vi "FOCUS_V42_H37.vi"(9 "X-pixels":sgl=256.0, 11 "Run":bool) -> (0 "Retrace pixels":sgl, 10 "Pixel Clock (Hz)":sgl)   [LabVIEW 2010] (continued)
                frame 2 {
                  # "line scan FScope"
                  n3346 = local read "LS X/Y"() -> (w6475:bool)
                  n3347 = case shown="True" w6475 {
                    tunnel: [w6513 w6514] -> w6476
                    frame False {
                      n3348 = local read "Y dim"() -> (w6513:sgl)
                    }
                    frame True {
                      n3349 = local read "X dim"() -> (w6514:sgl)
                    }
                  }
                  n3350 = Initialize Array(u32 0 ("element"), w6476) -> (w6477:u32[])
                  n3351 = Unbundle By Name(w6497) -> ("status"=w6495:bool)
                  n3352 = Unbundle By Name(w6493) -> ("status"=w6492:bool)
                  n3353 = Unbundle By Name(w6496) -> ("status"=w6494:bool)
                  n3354 = while {
                    tunnel: w6506 -> [w6586]
                    tunnel: w6505 -> [w6585]
                    tunnel: [w6584] -> w6504
                    tunnel: [w6576] -> w6503
                    shift-right: [w6524] -> w6473
                    shift-left: w6498 -> [w6536]
                    shift-right: [w6526] -> w6472
                    shift-left: w6498 -> [w6535]
                    tunnel: [w6580] -> w6500
                    tunnel: w6502 -> [w6580]
                    tunnel: [w6577] -> w6499
                    tunnel: w6501 -> [w6577]
                    shift-right: [w6530] -> _
                    shift-left: w6477 -> [w6519]
                    tunnel: w6495 -> [w6573]
                    tunnel: w6494 -> [w6578]
                    tunnel: w6492 -> [w6561]
                    shift-right: [w6567] -> _
                    shift-left: sgl 0.0 ("millisecond timer value") -> [w6570]
                    tunnel: w6490 -> [w6566]
                    tunnel: w6487 -> [w6564]
                    tunnel: [w6564] -> w6485
                    tunnel: [w6563] -> w6484
                    tunnel: w6486 -> [w6563]
                    tunnel: w6483 -> [w6529]
                    shift-right: [w6551] -> _
                    shift-left: w6481 -> [w6553]
                    shift-right: [w6549] -> _
                    shift-left: w6482 -> [w6550]
                    tunnel: w6475 -> [w6533]
                    tunnel: [w6522] -> w6474
                    i -> [w6528]
                    stop <- w6572 stop-if-true
                    n3355 = local read "ScaleCluster"() -> (w6559:T3)
                    n3356 = local read "Overlay Images"() -> (w6581:bool)
                    n3357 = Bundle("ScaleCluster"=w6559, "scans to read"=w6529) -> (w6551:T20)  [unwired: 1 in]
                    n3358 = call-poly <vilib>:"DAQmx Read (Digital 1D U32 1Chan NSamp).vi"("task/channels in"=w6586, "number of samples per channel"=w6529, "error in"=w6585) -> ("task out"=w6584:refnum<k21>, "data"=w6517:u32[], "error out"=w6576:errorcluster)  [unwired: 10 in]
                    n3359 = Not Equal?(x=w6551, y=w6553) -> (x != y?=w6552:bool)
                    n3360 = Multiply(x=u32 0 ("millisecond timer value"), y=w6519) -> (x*y=w6518:u32[])
                    n3361 = call-poly <vilib>:"Ramp Pattern.vi"("start"=0.0, "end"=6.283185307179586, "samples"=w6529) -> ("Ramp Pattern"=w6548:dbl[])  [unwired: 7 in, 1 out]
                    n3362 = case shown="False" w6552 {
                      tunnel: w6566 -> [_ w6592]
                      tunnel: [w6589 w6591] -> w6549
                      tunnel: w6551 -> [_ w6590]
                      tunnel: w6550 -> [w6589 _]
                      frame False {
                      }
                      frame True {
                        n3363 = call "ScaleScanlineFScope.vi"("Parameters"=w6592, "ScaleCluster"=w6590) -> ("ScanlineScaled"=w6591:dbl[][])
                      }
                    }
                    n3364 = Split Number(x=w6517) -> (hi(x)=w6583:u16[])  [unwired: 1 out]
                    n3365 = Sine(x=w6548) -> (sin(x)=w6546:dbl[])
                    n3366 = Split Number(x=w6583) -> (hi(x)=w6521:u8[], lo(x)=w6582:u8[])
                    n3367 = case shown="True" w6581 {
                      tunnel: w6521 -> [w6598 w6617]
                      tunnel: [w6598 w6600] -> w6534
                      tunnel: w6582 -> [w6597 w6619]
                      tunnel: [w6597 _] -> w6531
                      frame False {
                      }
                      frame True {
                        n3368 = To Word Integer(number=w6617) -> (16bit integer=w6618:i16[])
                        n3369 = Subtract(x=w6618, y=w6619) -> (x-y=w6599:i16[])
                        n3370 = Add(x=w6618, y=w6619) -> (x+y=w6613:i16[])
                        n3371 = Increment(x=w6613) -> (x+1=w6623:i16[])
                        n3372 = Divide(x=w6599, y=w6623) -> (x/y=w6622:dbl[])
                        n3373 = Absolute Value(x=w6599) -> (abs(x)=w6615:i16[])
                        n3374 = Multiply(x=w6622, y=u8 2) -> (x*y=w6620:dbl[])
                        n3375 = Round To Nearest(number=w6620) -> (nearest integer value=w6606:dbl[])
                        n3376 = Divide(x=w6615, y=2.0) -> (x/y=w6612:dbl[])
                        n3377 = Divide(x=w6613, y=2.0) -> (x/y=w6611:dbl[])
                        n3378 = Add(x=w6612, y=w6611) -> (x+y=w6609:dbl[])
                        n3379 = Divide(x=w6609, y=5.0) -> (x/y=w6608:dbl[])
                        n3380 = Round To Nearest(number=w6608) -> (nearest integer value=w6607:dbl[])
                        n3381 = Multiply(x=5.0 ("y"), y=w6607) -> (x*y=w6605:dbl[])
                        n3382 = Add(x=w6606, y=w6605) -> (x+y=w6604:dbl[])
                        n3383 = Subtract(x=w6604, y=2.0) -> (x-y=w6601:dbl[])
                        n3384 = To Unsigned Byte Integer(number=w6601) -> (unsigned 8bit integer=w6600:u8[])
                      }
                    }
                    n3385 = Add(x=w6546, y=sgl 2.0 ("millisecond timer value")) -> (x+y=w6541:dbl[])
                    n3386 = Divide(x=u32 4294967295 ("millisecond timer value"), y=sgl 3.0) -> (x/y=w6542:sgl)
                    n3387 = Array Subset(array=w6549, index (col)=w6570, length (col)=w6529) -> (w6532:dbl[][])  [unwired: 2 in]
                    n3388 = Multiply(x=w6542, y=w6541) -> (x*y=w6540:dbl[])
                    n3389 = To Unsigned Long Integer(number=w6540) -> ()  [unwired: 1 out]
                    n3390 = Index Array(array=w6549, index (row)=0) -> (element=w6557:dbl[])  [unwired: 1 in]
                    n3391 = Array Size(array=w6557) -> (size(s)=w6555:i32)
                    n3392 = Divide(x=w6555, y=2) -> (x/y=w6554:dbl)
                    n3393 = Add(x=w6570, y=w6529) -> (x+y=w6568:dbl)
                    n3394 = local read "LS X/Y"() -> (w6538:bool)
                    n3395 = Greater Or Equal?(x=w6568, y=w6554) -> (x >= y?=w6569:bool)
                    n3396 = case shown="False" w6538 {
                      tunnel: [w6587 w6588] -> w6537
                      frame False {
                        n3397 = local read "X dim"() -> (w6587:sgl)
                      }
                      frame True {
                        n3398 = local read "Y dim"() -> (w6588:sgl)
                      }
                    }
                    n3399 = case shown="True" w6569 {
                      tunnel: w6568 -> [w6593 w6596]
                      tunnel: [w6593 w6594] -> w6567
                      tunnel: w6554 -> [_ w6595]
                      frame False {
                      }
                      frame True {
                        n3400 = Subtract(x=w6596, y=w6595) -> (x-y=w6594:dbl)
                      }
                    }
                    n3401 = Decrement(x=w6537) -> (x-1=w6562:sgl)
                    n3402 = Equal?(x=w6562, y=w6528) -> (x = y?=w6560:bool)
                    n3403 = call "AverageImageLSFScope.vi"("Index"=w6528, "ScanLineFScope"=w6532, "DataImage2"=w6531, "DataImage1"=w6534, "Image2Array"=w6535, "LS X/Y"=w6533, "Image1Array"=w6536, "HitsArrayLS"=w6518) -> ("Image2Arraynew"=w6526:u8[][], "Image1Arraynew"=w6524:u8[][], "HitsArrayLSnew"=w6530:u32[])
                    n3404 = local read "X dim"() -> (w6527:sgl)
                    n3405 = Build Array(w6530) -> (w6516:u32[][])
                    n3406 = Subtract(x=w6528, y=w6527) -> (x-y=w6522:sgl)
                    n3407 = Transpose 2D Array(2D array=w6516) -> (transposed array=w6515:u32[][])
                    n3408 = Array Subset(array=w6526, index (col)=w6522, length (col)=w6527) -> (w6525:u8[][])  [unwired: 2 in]
                    n3409 = local write "Hit Graph"(w6515) -> ()
                    n3410 = Array Subset(array=w6524, index (col)=w6522) -> (w6523:u8[][])  [unwired: 3 in]
                    n3411 = local write "Image 2"(w6525) -> ()
                    n3412 = local write "Image 1"(w6523) -> ()
                    n3413 = Unbundle By Name(w6563) -> ("status"=w6565:bool)
                    n3414 = Unbundle By Name(w6576) -> ("status"=w6574:bool)
                    n3415 = Unbundle By Name(w6577) -> ("status"=w6575:bool)
                    n3416 = local read "stop 2"() -> (w6579:bool)
                    n3417 = local read "End experiment"() -> (w6571:bool)
                    n3418 = Compound Arithmetic op=OR(w6579, w6578, w6575, w6574, w6573, w6565, w6560, w6561, w6571) -> (w6572:bool)
                  }
                }
              }
            }
          }
          "ScanLineLength" <- w3422
          "ZSinLength" <- w3421
          "DataOffset" <- w3420
          n3419 = Round Toward +Infinity(x=w3377) -> (ceil(x): smallest int >= x=w3379:sgl)
          n3420 = property on="ImageSlide" class="Slide (strict)"("Scale.Range:Minimum"=0.0, "Scale.Range:Maximum"=w3377) -> ()  [unwired: 2 in, 2 out]
          n3421 = local write "ImageSlide"(w3379) -> ()
          n3422 = Equal?(x=w3403, y=w3402) -> (x = y?=w3391:bool)
          n3423 = Multiply(x=sgl 1000.0, y="Time interval [s]") -> (x*y=w3312:sgl)
          n3424 = Not(x=w3400) -> (.not. x?=w3390:bool)
          n3425 = local read "Zsin3D"() -> (w3322:sgl[])
          n3426 = Subtract(x=w3312, y=w3364) -> ()  [unwired: 1 out]
          n3427 = In Range and Coerce(upper limit=w3312, x=w3312, lower limit=sgl 0.0) -> (coerced(x)=w3362:sgl)  [unwired: 1 out]
          n3428 = Array Size(array=w3339) -> (size(s)=w3338:i32[])
          n3429 = Array Size(array=w3336) -> (size(s)=w3337:i32[])
          n3430 = Or(x=w3390, y=w3391) -> (x .or. y?=w3392:bool)
          n3431 = local read "frame/line indicator"() -> (w3325:u16)
          n3432 = Multiply Array Elements(1:w3338) -> (0:w3335:i32)
          n3433 = Multiply Array Elements(1:w3337) -> (0:w3334:i32)
          n3434 = Unbundle(w3343) -> ("Output: VISA session OUT"=w3347:refnum<visa-resource-name>, "Error cluster"=w3346:errorcluster)
          n3435 = Index Array(array=w3321, index (row)=0 ("disabled index (col)")) -> (element=w3316:sgl[])  [unwired: 1 in]
          n3436 = Index Array(array=w3321, index (row)=1 ("disabled index (col)")) -> (element=w3315:sgl[])  [unwired: 1 in]
          n3437 = Add(x=w3335, y=w3334) -> (x+y=w3333:i32)
          "DataLength" <- w3333
          n3438 = property class="Serial Instr"(reference=w3347, error in=w3346) -> (reference out=w3348:refnum<visa-resource-name>, error out=w3349:errorcluster, "Serial Settings:Number of Bytes at Serial Port"=w3350:u32)
          n3439 = Interleave 1D Arrays(w3316, w3315, w3322) -> (w3320:sgl[])
          n3440 = local read "Positions"() -> (w3314:sgl[])
          n3441 = Greater Than 0?(x=w3325) -> (x > 0?=w3324:bool)
          n3442 = Greater Or Equal?(x=w3325, y=u16 3) -> (x >= y?=w3327:bool)
          n3443 = Array Size(array=w3320) -> (size(s)=w3319:i32)
          n3444 = property on="Property Node" class="VI"() -> ("VI Path"=w3328:path)  [unwired: 2 in, 2 out]
          n3445 = Build Array (concatenate)(w3319, w3320, w3314) -> (w3313:sgl[])
          n3446 = VISA Read(VISA resource name=w3348, byte count=w3350, error in (no error)=w3349) -> (VISA resource name out=w3344:refnum<visa-resource-name>, error out=w3345:errorcluster)  [unwired: 2 out]
          n3447 = case shown="True" w3324 {
            tunnel: w3327 -> [_ w3445]
            tunnel: w3328 -> [_ w3444]
            tunnel: w3323 -> [_ w3443]
            tunnel: w3313 -> [_ w3442]
            frame False {
            }
            frame True {
              n3448 = case shown="True" "Autosave" {
                tunnel: w3445 -> [_ w3451]
                tunnel: w3443 -> [_ w3449]
                tunnel: w3444 -> [_ w3448]
                tunnel: w3442 -> [_ w3447]
                frame False {
                }
                frame True {
                  n3449 = local read "FilePath"() -> (w3453:path)
                  n3450 = local read "BaseFilename"() -> (w3452:string)
                  n3451 = Bundle("BaseFilename"=w3452, "FilePath"=w3453, "Autoincrement\nFilename"=TRUE ("Autoincrement\nFilename"), w3451) -> (w3450:T35)  [unwired: 1 in]
                  n3452 = call "SavenewFOCUS.vi"("source path"=w3448, "Header"=w3449, "Positions"=w3447, "Parameters"=w3450) -> ("Data directory out"=w3455:path, "name"=w3457:string, "basename out"=w3456:string)
                  n3453 = local write "Save?"(TRUE ("Save?")) -> ()
                  n3454 = local write "BaseFilename"(w3456) -> ()
                  n3455 = local write "FilePath"(w3455) -> ()
                  n3456 = local write "Filename"(w3457) -> ()
                }
              }
            }
          }
          n3457 = local read "Sutter scale x"() -> (w3301:sgl)
          n3458 = local read "Sutter scale y"() -> (w3300:sgl)
          n3459 = local read "Sutter scale z"() -> (w3299:sgl)
          n3460 = Bundle("Output: VISA session OUT"=w3344, "error out"=w3345) -> (w3342:T36)  [unwired: 1 in]
          n3461 = call "VISA MP-285 Get Position.vi"("Input: Duty Cluster"=w3342) -> ("Output: X axis (microns)"=w3358:dbl, "Output: Y axis (microns)"=w3357:dbl, "Output: Z axis (microns)"=w3356:dbl, "Output: Duty Cluster"=w3352:T18)
          n3462 = case shown="False" w3392 {
            tunnel: [w6682 w6706] -> w3384
            tunnel: w3352 -> [w6681 w6708]
            tunnel: [w6680 w6708] -> w3351
            tunnel: [w6679 w6705] -> w3398
            tunnel: w3396 -> [w6678 w6706]
            tunnel: w3395 -> [w6677 w6705]
            tunnel: w3387 -> [w6676 w6707]
            tunnel: w3394 -> [w6675 w6709]
            tunnel: [w6674 w6709] -> w3393
            tunnel: w3362 -> [w6673 _]
            tunnel: [w6672 w6707] -> w3386
            frame False {
              n3463 = local read "Number of frames"() -> (w6668:sgl)
              n3464 = flat-sequence {
                tunnel: w6673 -> [w6694]
                tunnel: [w6694] -> w6688
                tunnel: [w6690] -> w6687
                tunnel: [w6689] -> w6686
                tunnel: w6678 -> [w6692]
                tunnel: w6677 -> [w6691]
                tunnel: [w6701] -> w6685
                tunnel: [w6700] -> w6684
                tunnel: [w6699] -> w6683
                tunnel: w6688 -> [w6701]
                tunnel: w6687 -> [w6700]
                tunnel: w6686 -> [w6699]
                tunnel: w6676 -> [w6698]
                tunnel: w6675 -> [w6697]
                tunnel: [w6696] -> w6674
                tunnel: [w6695] -> w6672
                tunnel: [w6704] -> w6682
                tunnel: [w6703] -> w6679
                tunnel: w6685 -> [w6702]
                tunnel: w6684 -> [w6704]
                tunnel: w6683 -> [w6703]
                frame #0 {
                  w6693 = FALSE ("data")
                  n3465 = local write "Shutter open"(w6693) -> ()
                  n3466 = call-poly <vilib>:"DAQmx Write (Digital Bool 1Line 1Point).vi"("task/channels in"=w6692, "data"=w6693, "error in"=w6691) -> ("task out"=w6690:refnum<k21>, "error out"=w6689:errorcluster)  [unwired: 10 in, 1 out]
                }
                frame #1 {
                  n3467 = call <vilib>:"DAQmx Stop Task.vi"("task/channels in"=w6698, "error in"=w6697) -> ("task out"=w6695:refnum<k21>, "error out"=w6696:errorcluster)  [unwired: 12 in]
                }
                frame #2 {
                  n3468 = Wait (ms)(milliseconds to wait=w6702) -> ()  [unwired: 1 out]
                }
              }
              n3469 = local read "z-step (um)"() -> (w6670:sgl)
              n3470 = local read "Sutter scale z"() -> (w6666:sgl)
              n3471 = Decrement(x=w6668) -> (x-1=w6667:sgl)
              n3472 = Multiply(x=w6670, y=w6667) -> (x*y=w6669:sgl)
              n3473 = Negate(x=w6666) -> (-x=w6665:sgl)
              n3474 = Divide(x=w6669, y=w6665) -> (x/y=w6671:sgl)
              n3475 = call "VISA MP-285 Step.vi"("Input: Duty Cluster"=w6681, "Input: Delta Z axis (microns)"=w6671) -> ("Output: Duty Cluster"=w6680:T18)  [unwired: 2 in, 3 out]
            }
            frame True {
            }
          }
          n3476 = Multiply(x=w3358, y=w3301) -> (x*y=→"x-positionstop (um)":dbl)
          n3477 = Multiply(x=w3357, y=w3300) -> (x*y=→"y-positionstop (um)":dbl)
          n3478 = Multiply(x=w3356, y=w3299) -> (x*y=→"z-positionstop (um)":dbl)
          n3479 = case shown="True" w3400 {
            tunnel: "Number of stacks" -> [_ w6727]
            tunnel: [TRUE w6722] -> w3399
            tunnel: w3402 -> [_ w6726]
            frame False {
            }
            frame True {
              n3480 = local read "End experiment"() -> (w6725:bool)
              n3481 = Increment(x=w6726) -> (x+1=w6721:i32)
              "#" <- w6721
              "#" <- w6721
              n3482 = local read "stop 2"() -> (w6724:bool)
              n3483 = Equal?(x=w6727, y=w6721) -> (x = y?=w6723:bool)
              n3484 = Compound Arithmetic op=OR(w6724, w6725, w6723) -> (w6722:bool)
            }
          }
          n3485 = case shown="True" w3399 {
            tunnel: w3398 -> [w6711 w6714]
            tunnel: [w6711 w6713] -> w3397
            tunnel: w3384 -> [w6710 w6715]
            tunnel: [w6710 w6712] -> w3383
            frame False {
            }
            frame True {
              w6716 = FALSE ("data")
              w6717 = u8 0 ("Disabled")
              w6718 = FALSE
              # "Sort out controls"
              n3486 = local write "stop 2"(w6718) -> ()
              n3487 = local write "Run"(w6718) -> ()
              n3488 = property on="Scan format" class="Ring (strict)"("Disabled"=w6717) -> ()  [unwired: 2 in, 2 out]
              n3489 = property on="X-pixels" class="DigNum (strict)"("Disabled"=w6717) -> ()  [unwired: 2 in, 2 out]
              n3490 = property on="Y-lines" class="DigNum (strict)"("Disabled"=w6717) -> ()  [unwired: 2 in, 2 out]
              n3491 = local write "Shutter open"(w6716) -> ()
              n3492 = call-poly <vilib>:"DAQmx Write (Digital Bool 1Line 1Point).vi"("task/channels in"=w6715, "data"=w6716, "error in"=w6714) -> ("task out"=w6712:refnum<k21>, "error out"=w6713:errorcluster)  [unwired: 10 in, 1 out]
              n3493 = property on="line scan time (ms)" class="DigNum (strict)"("Disabled"=w6717) -> ()  [unwired: 2 in, 2 out]
              n3494 = property on="Rotation" class="Knob (strict)"("Disabled"=w6717) -> ()  [unwired: 2 in, 2 out]
              n3495 = property on="Zoom" class="Slide (strict)"("Disabled"=w6717) -> ()  [unwired: 2 in, 2 out]
              n3496 = property on="Run" class="Bool (strict)"("Visible"=TRUE) -> ()  [unwired: 2 in, 2 out]
              n3497 = property on="Measurement cursor check box" class="Bool (strict)"("Disabled"=w6717) -> ()  [unwired: 2 in, 2 out]
              n3498 = property on="View line\ncheck box" class="Bool (strict)"("Disabled"=w6717) -> ()  [unwired: 2 in, 2 out]
            }
          }
        }
      }
    }
    "Image1Array" <- w191
    "Image2Array" <- w190
    "Image3Array" <- w189
    "Image4Array" <- w188
    n3499 = case shown="True" w210 {
      tunnel: w217 -> [_ w347]
      tunnel: w216 -> [_ w346]
      frame False {
      }
      frame True {
        n3500 = call <vilib>:"DAQmx Clear Task.vi"("task in"=w346, "error in"=w347) -> ("error out"=w348:errorcluster)  [unwired: 13 in]
        n3501 = call <vilib>:"Simple Error Handler.vi"("error in (no error)"=w348) -> ()  [unwired: 4 in, 5 out]
      }
    }
    n3502 = stacked-sequence {
      tunnel: [w349] -> w252
      tunnel: w224 -> [_]
      frame #0 {
        n3503 = local read "AO/DIO Device"() -> (w349:tag)
      }
    }
    n3504 = local read "frame/line indicator"() -> (w255:u16)
    n3505 = local read "frame/line indicator"() -> (w258:u16)
    n3506 = Unbundle(w199) -> ("Output: VISA session OUT"=w203:refnum<visa-resource-name>, "Error cluster"=w202:errorcluster)
    n3507 = call <vilib>:"DAQmx Clear Task.vi"("task in"=w270, "error in"=w271) -> ("error out"=w269:errorcluster)  [unwired: 13 in]
    n3508 = call <vilib>:"DAQmx Clear Task.vi"("task in"=w274, "error in"=w273) -> ("error out"=w275:errorcluster)  [unwired: 13 in]
    n3509 = call <vilib>:"DAQmx Clear Task.vi"("task in"=w267, "error in"=w266) -> ("error out"=w265:errorcluster)  [unwired: 13 in]
    n3510 = property class="Serial Instr"(reference=w203, error in=w202) -> (reference out=w204:refnum<visa-resource-name>, error out=w205:errorcluster, "Serial Settings:Number of Bytes at Serial Port"=w206:u32)
    n3511 = call <vilib>:"Simple Error Handler.vi"("error in (no error)"=w275) -> ()  [unwired: 4 in, 5 out]
    n3512 = call <vilib>:"Simple Error Handler.vi"("error in (no error)"=w269) -> ()  [unwired: 4 in, 5 out]
    n3513 = call <vilib>:"DAQmx Clear Task.vi"("task in"=w268, "error in"=w265) -> ("error out"=w263:errorcluster)  [unwired: 13 in]
    n3514 = Equal?(x=w255, y=u16 4) -> (x = y?=w166:bool)
    n3515 = Concatenate Strings(tag "/" ("destination terminal"), w252) -> (w228:string)
    n3516 = Concatenate Strings(w228, tag "/PXI_Trig2" ("source terminal")) -> (w239:string)
    n3517 = Concatenate Strings(w228, tag "/PFI2" ("destination terminal")) -> (w241:string)
    n3518 = Concatenate Strings(w228, tag "/PXI_Trig2" ("destination terminal")) -> (w248:string)
    n3519 = Concatenate Strings(w228, tag "/10MHzRefClock" ("source terminal")) -> (w251:string)
    n3520 = Type Cast(type=tag "" ("destination terminal"), x=w239) -> (*(type *) &x=w237:tag)
    n3521 = Type Cast(type=tag "" ("destination terminal"), x=w241) -> (*(type *) &x=w236:tag)
    n3522 = Type Cast(type=tag "" ("destination terminal"), x=w248) -> (*(type *) &x=w244:tag)
    n3523 = Type Cast(type=tag "" ("destination terminal"), x=w251) -> (*(type *) &x=w245:tag)
    n3524 = call <vilib>:"DAQmx Disconnect Terminals.vi"("source terminal"=w245, "destination terminal"=w244, "error in"=w280) -> ("error out"=w281:errorcluster)  [unwired: 12 in]
    n3525 = Greater Or Equal?(x=w258, y=u16 3) -> (x >= y?=w256:bool)
    n3526 = call <vilib>:"Simple Error Handler.vi"("error in (no error)"=w263) -> ()  [unwired: 4 in, 5 out]
    n3527 = Or(x=w166, y=w164) -> (x .or. y?=w165:bool)
    n3528 = VISA Read(VISA resource name=w204, byte count=w206, error in (no error)=w205) -> (VISA resource name out=w200:refnum<visa-resource-name>, error out=w201:errorcluster)  [unwired: 2 out]
    n3529 = case shown="True" w256 {
      tunnel: w272 -> [_ w354]
      tunnel: w224 -> [_ w353]
      frame False {
      }
      frame True {
        n3530 = call <vilib>:"DAQmx Clear Task.vi"("task in"=w354, "error in"=w353) -> ("error out"=w355:errorcluster)  [unwired: 13 in]
        n3531 = call <vilib>:"Simple Error Handler.vi"("error in (no error)"=w355) -> ()  [unwired: 4 in, 5 out]
      }
    }
    n3532 = call <vilib>:"DAQmx Disconnect Terminals.vi"("source terminal"=w237, "destination terminal"=w236, "error in"=w281) -> ("error out"=w235:errorcluster)  [unwired: 12 in]
    n3533 = Concatenate Strings(w228, tag "/PFI5" ("destination terminal")) -> (w232:string)
    n3534 = case shown="False" w165 {
      tunnel: w294 -> [w352 _]
      tunnel: w293 -> [w351 _]
      frame False {
        n3535 = call <vilib>:"DAQmx Clear Task.vi"("task in"=w351, "error in"=w352) -> ("error out"=w350:errorcluster)  [unwired: 13 in]
        n3536 = call <vilib>:"Simple Error Handler.vi"("error in (no error)"=w350) -> ()  [unwired: 4 in, 5 out]
      }
      frame True {
      }
    }
    n3537 = Concatenate Strings(w228, tag "/ao/SampleClock" ("source terminal")) -> (w229:string)
    n3538 = Type Cast(type=tag "" ("destination terminal"), x=w232) -> (*(type *) &x=w227:tag)
    n3539 = Bundle("Output: VISA session OUT"=w200, "error out"=w201) -> (w162:T36)  [unwired: 1 in]
    n3540 = Type Cast(type=tag "" ("destination terminal"), x=w229) -> (*(type *) &x=w226:tag)
    n3541 = call <vilib>:"DAQmx Disconnect Terminals.vi"("source terminal"=w226, "destination terminal"=w227, "error in"=w235) -> ("error out"=w225:errorcluster)  [unwired: 12 in]
    n3542 = call <vilib>:"DAQmx Clear Task.vi"("task in"=w278, "error in"=w225) -> ("error out"=w279:errorcluster)  [unwired: 13 in]
    n3543 = call <vilib>:"Simple Error Handler.vi"("error in (no error)"=w279) -> ()  [unwired: 4 in, 5 out]
    "Line Clock" <- w298
    "Frame Clock" <- w262
    "Position Signals" <- w261
    "Scan Signals" <- w260
    "Data Input" <- w259
  }
  n3544 = flat-sequence {
    tunnel: [w6799] -> w6
    tunnel: w4 -> [_]
    frame #0 {
      w6802 = "L"  # Resolution (L or H)
      n3545 = Type Cast(type=" ", x="VISA Sutter MP-285") -> (*(type *) &x=w6807:string)
      n3546 = Reverse String(1:w6807) -> (0:w6806:string)
      n3547 = String Subset(string=w6806, offset (0)=0, length (rest)=1 ("length (rest)")) -> (substring=w6803:string)
      n3548 = Decimal String To Number(string=w6803) -> (number=w6810:i32)  [unwired: 2 in, 1 out]
      n3549 = local read "Sutter Speed [um/s]"() -> (w6798:i32)
      n3550 = call "VISA MP-285 InitNotRefresh.vi"("baud rate (9600)"=u32 9600, "Timeout (msec)"=u32 700, "Serial port # \n(COM1 - #1)!!!"=w6810) -> ("Output: Duty Cluster"=w6801:T18)  [unwired: 1 in]
      n3551 = call "VISA MP-285 GetSet Resolution.vi"("Input: Resolution - H/L"=w6802, "Input: Duty Cluster"=w6801) -> ("Output: Duty Cluster"=w6800:T18)  [unwired: 2 out]
      n3552 = Add(x=w6798, y=300) -> (x+y=w6796:i32)
      n3553 = call "VISA MP-285 GetSet Speed.vi"("Input: Duty Cluster"=w6800, "Input: Speed in microns/sec"=w6796) -> ("Output: Duty Cluster"=w6799:T18)  [unwired: 1 out]
    }
  }
  n3554 = call "VISA MP-285 Close.vi"("Input: Duty Cluster"=w5) -> ()  [unwired: 1 out]
  "Program Version" <- w87
